vi "E_turbo_pump_status.vi"(3 "error in":errorcluster, 4 "task/channels in":refnum<k21>, 5 "test mode":bool, 6 "test value":bool) -> (0 "error out":errorcluster, 1 "element":bool)   [LabVIEW 2013]
uses:
  <vilib>/DAQmx/read.llb/DAQmx Read (Digital 1D Bool NChan 1Samp 1Line).vi
  <vilib>/DAQmx/miscellaneous.llb/DAQmx Fill In Error Info.vi
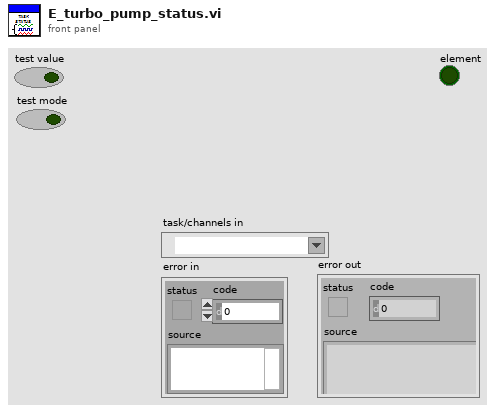
[diagram p1: front panel]
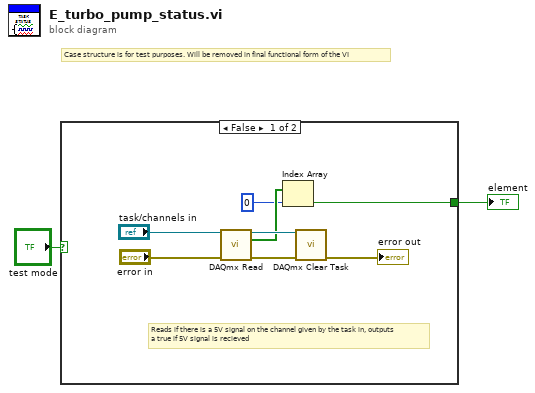
[diagram p0: block diagram]
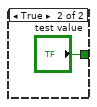
[diagram p2: hidden frame]
diagram:
  # "Case structure is for test purposes. Will be removed in final functional form of the VI"
  n1 = case shown="False" "test mode" {
    tunnel: [w3 "test value"] -> w2
    frame False {
      # "Reads if there is a 5V signal on the channel given by the task in, outputs\na true if 5V signal is recieved"
      n2 = call-poly <vilib>:"DAQmx Read.vi"("task/channels in"="task/channels in", "error in"="error in") -> ("task out"=w9:refnum<k21>, "data"=w6:bool[], "error out"=w10:errorcluster)  [unwired: 11 in]
      n3 = Index Array(array=w6, index=0) -> (element=w3:bool)
      n4 = call <vilib>:"DAQmx Clear Task.vi"("task in"=w9, "error in"=w10) -> ("error out"=→"error out":errorcluster)  [unwired: 13 in]
    }
    frame True {
    }
  }
  "element" <- w2
